vi "Get_Score_Info_Web.vi"(8 "LabVIEW Web Service Request":refnum<class "Web Request.lvclass">, 10 "Round":u16, 11 "Team":u16) -> ()   [LabVIEW 2013]
uses:
  <vilib>/wsapi/Web Request.lvclass
  <vilib>/xml/Close Reference(Node).vi
  <vilib>/xml/NI_XML.lvlib
  <resource>/objmgr/DOMUserDefRef.rc
panel:
  out "XML":string
  in  "Web?":bool=TRUE
  out "Score Data":cluster{"Tag":string, "Value":string}[](array[cluster])
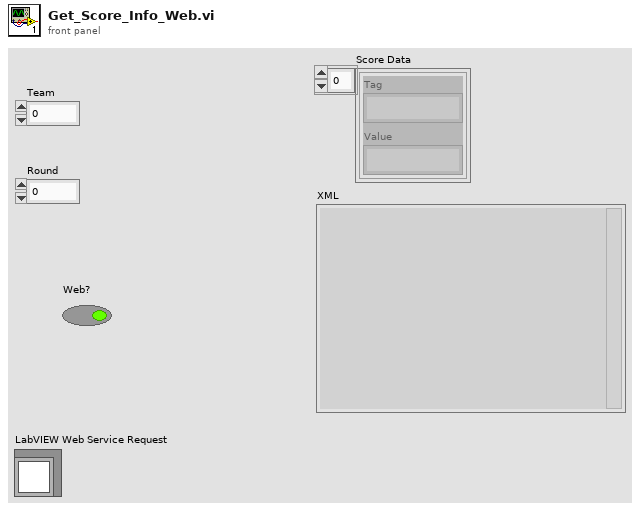
[diagram p1: front panel]
types:
  T1 = typedef "Team Data.ctl" = cluster{"Both":string, "Name":string, "GUID":u16, "Number":u16}
  T2 = typedef "ScoreList.ctl" = cluster{"ValidationCount":u16, "Score":T3}[]
  T3 = typedef "Full Score Entry.ctl" = cluster{"GUID":u16, "Score Mode Selector":u16, "Round Number":u16, "Full Score Entry":T4}
  T4 = typedef "ScoreEntry.ctl" = cluster{"Elements":cluster{"Name":string, "Value":string}[], "Score":dbl}
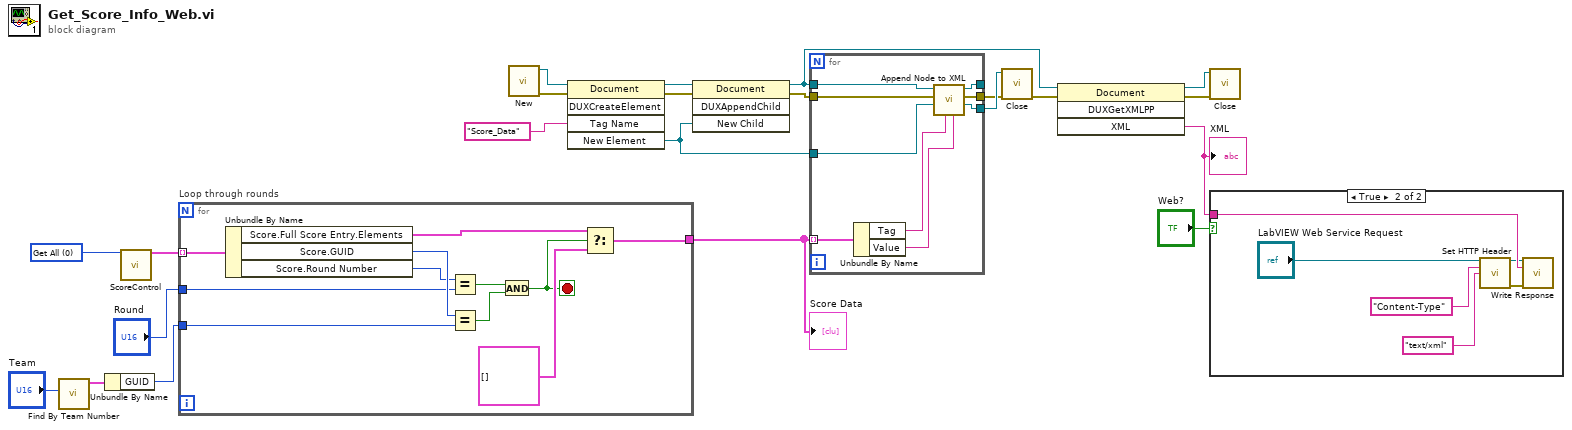
[diagram p0: block diagram]
diagram:
  w5 = u16 0 items=["Get All", "Set", "Reset All", "Force Set"] ("Get/Set Mode Selector")
  n1 = call "Find By Team Number.vi"("Team Number"="Team") -> ("Team Data"=w2:T1)  [unwired: 9 in, 1 out]
  n2 = Unbundle By Name(w2) -> ("GUID"=w1:u16)
  n3 = call "ScoreControl.vi"("Get/Set Mode Selector"=w5) -> ("Scores"=w4:T2)  [unwired: 13 in, 1 out]
  n4 = for "Loop through rounds" {
    tunnel: w4 -> [w25] mode=indexing
    tunnel: "Round" -> [w29]
    tunnel: [w33] -> w21
    tunnel: w1 -> [w23]
    stop <- w26 stop-if-true
    n5 = Unbundle By Name(w25) -> ("Score.Full Score Entry.Elements"=w24:cluster{"Name":string, "Value":string}[], "Score.GUID"=w31:u16, "Score.Round Number"=w30:u16)
    n6 = Equal?(x=w30, y=w29) -> (x = y?=w28:bool)
    n7 = Equal?(x=w31, y=w23) -> (x = y?=w27:bool)
    n8 = And(x=w28, y=w27) -> (x .and. y?=w26:bool)
    n9 = Select(t=w24, s=w26, f=cluster{"Tag":string, "Value":string}[] []) -> (s? t:f=w33:cluster{"Tag":string, "Value":string}[])
  }
  "Score Data" <- w21
  n10 = call <vilib>:"New.vi"() -> ("error out"=w19:errorcluster, "DOM document out"=w20:refnum<k20>)  [unwired: 8 in]
  n11 = invoke class="Document" method="DUXCreateElement"(reference=w20, error in=w19, "Tag Name"="Score_Data") -> (reference out=w17:refnum<k20>, error out=w16:errorcluster, "New Element"=w14:refnum<k20>)  [unwired: 2 in, 2 out]
  n12 = invoke class="Document" method="DUXAppendChild"(reference=w17, error in=w16, "New Child"=w14) -> (reference out=w7:refnum<k20>, error out=w15:errorcluster)  [unwired: 1 in, 2 out]
  n13 = for {
    tunnel: w21 -> [w40] mode=indexing
    tunnel: w7 -> [w42]
    tunnel: w15 -> [w41]
    tunnel: w14 -> [w36]
    tunnel: [w39] -> _
    tunnel: [w38] -> w10
    tunnel: [w37] -> w11
    n14 = Unbundle By Name(w40) -> ("Tag"=w34:string, "Value"=w35:string)
    n15 = call "Append Node to XML.vi"("Data"=w35, "Tag Name"=w34, "SuperElement In"=w36, "error in"=w41, "DOM document in"=w42) -> ("SuperElement Out"=w37:refnum<k20>, "error out"=w38:errorcluster, "DOM document out"=w39:refnum<k20>)  [unwired: 4 in]
  }
  n16 = call-poly <vilib>:"Close.vi"("error in (no error)"=w10, "node"=w11) -> ("error out"=w6:errorcluster)  [unwired: 7 in]
  n17 = invoke class="Document" method="DUXGetXMLPP"(reference=w7, error in=w6) -> (reference out=w13:refnum<k20>, error out=w12:errorcluster, "XML"=w9:string)  [unwired: 2 in, 1 out]
  "XML" <- w9
  n18 = call-poly <vilib>:"Close.vi"("error in (no error)"=w12, "node"=w13) -> ()  [unwired: 7 in, 1 out]
  n19 = case shown="True" "Web?" {
    tunnel: w9 -> [_ w48]
    frame False {
    }
    frame True {
      n20 = call <vilib>:"Set HTTP Header.vi"("LabVIEW Web Service Request"="LabVIEW Web Service Request", "header"="Content-Type", "header value"="text/xml") -> ("LabVIEW Web Service Request out"=w44:refnum<class "Web Request.lvclass">, "error out"=w43:errorcluster)  [unwired: 11 in]
      n21 = call <vilib>:"Write Response.vi"("LabVIEW Web Service Request"=w44, "response string"=w48, "error in (no error)"=w43) -> ()  [unwired: 11 in, 2 out]
    }
  }
